vi "CODMn通讯.vi"() -> ()   [LabVIEW 2016, in "斯坦道CODMn.lvlib"]
uses:
  <vilib>/Utility/error.llb/DialogType.ctl
  <vilib>/NI/Modbus Library/API/Wrapper/Create TCP Slave.vi
  <vilib>/NI/Modbus Library/API/slave/Modbus Slave.lvclass
  <vilib>/Plasmionique/MB Master/MB_Master/MB_Master.lvclass
  <vilib>/Plasmionique/MB Master/MB Master.lvlib
  <vilib>/Utility/config.llb/NI_LVConfig.lvlib
  <vilib>/NI/Modbus Library/API/Wrapper/API Main.lvlib
panel:
  out "codm程序更新":bool=TRUE
  in  "读取数据":bool
  in  "释放串口":bool
  in  "打开串口":bool
  out "队列中元素数量":i32
  out "元素":cluster{"命令":string}[](array[cluster])
  out "待处理插入数量":i32
  out "读取公式":u16[](array[numeric])
  out "读取参数":u16[](array[numeric])
  out "数据存储":u16[](array[numeric])
  out "温度":bool[](array[boolean])
  out "M输出点":bool[](array[boolean])
  out "ORP、时间":u16[](array[numeric])
  out "测量状态":u16[](array[numeric])
  out "通讯状态":bool
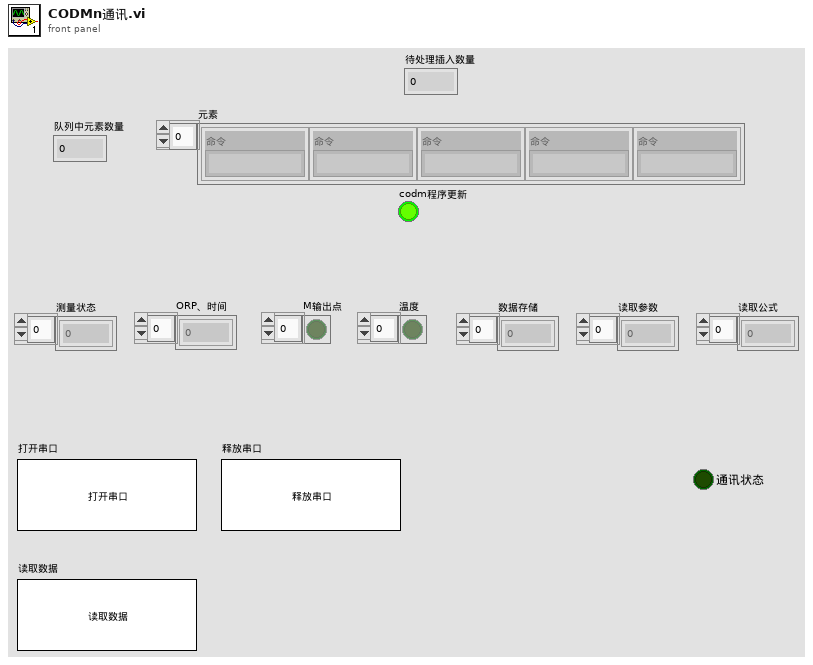
[diagram p1: front panel]
types:
  T1 = typedef "CODMn交互.ctl" = cluster{"COD浓度（mg/L)":dbl, "水样启动时间":timestamp, "加标回收启动时间":timestamp, "CODMn工作状态":enum16{"空闲", "水样测试", "标样核查", "零点核查", "跨度核查", "空白测试", "平行样测试", "加标回收", "空白校准", "标样校准", "初始化（清洗）"}, "多列列表框":i32, "平台试剂余量百分比":sgl, "关键参数":cluster{"测量量程":dbl, "测量精度":dbl, "测量间隔":dbl, "消解温度":dbl, "消解时长":dbl, "空白校准时间":timestamp, "曲线截距":dbl, "曲线斜率":dbl, "测量检出限":dbl, "测量信号值":dbl, "线性相关系数":dbl, "二次多项式系数":dbl, "标样校准时间":timestamp, "稀释倍数":dbl, "三项式系数":dbl, "空白标定系数":dbl, "量程系数":dbl, "F0/ORPA":dbl, "F1/ORPB":dbl, "F2/ORPK":dbl, "F3":dbl, "F4":dbl, "F5":dbl, "F6":dbl, "F7":dbl, "X0/滴定数":dbl, "量程":dbl}, "关键参数改变":bool, "校准信息":cluster{"低标液1浓度":dbl, "低标液1信号值":dbl, "低标液1启用":u16, "低标液2浓度":dbl, "低标液2信号值":dbl, "低标液2启用":u16, "低标液3浓度":dbl, "低标液3信号值":dbl, "低标液3启用":u16, "低标液4浓度":dbl, "低标液4信号值":dbl, "低标液4启用":u16, "低标液5浓度":dbl, "低标液5信号值":dbl, "低标液5启用":u16, "高标液1浓度":dbl, "高标液1信号值":dbl, "高标液1启用":u16, "高标液2浓度":dbl, "高标液2信号值":dbl, "高标液2启用":u16, "高标液3浓度":dbl, "高标液3信号值":dbl, "高标液3启用":u16, "高标液4浓度":dbl, "高标液4信号值":dbl, "高标液4启用":u16, "高标液5浓度":dbl, "高标液5信号值":dbl, "高标液5启用":u16}, "校准信息改变":bool}
  T2 = cluster{"测量模式":enum16{"水样测量", "标样核查", "零点核查", "跨度核查", "空白测试", "加标回收", "平行样", "校零", "校标"}}
  T3 = cluster{"命令":string, "测量模式":enum16{"水样测量", "标样核查", "零点核查", "跨度核查", "空白测试", "加标回收", "平行样", "校零", "校标"}, "CODMn量程切换":enum32{"H", "L", "AUTO"}}
  T4 = typedef "NI_LVConfig.lvlib/Config Data RefNum.ctl" = refnum<k1>
  T5 = enum16{"空闲", "水样测试", "标样核查", "零点核查", "跨度核查", "空白测试", "平行样测试", "质控样", "空白校准", "标样校准", "加标回收"}
  T6 = cluster{"测量量程":dbl, "测量精度":dbl, "测量间隔":dbl, "消解温度":dbl, "消解时长":dbl, "空白校准时间":timestamp, "曲线截距":dbl, "曲线斜率":dbl, "测量检出限":dbl, "测量信号值":dbl, "线性相关系数":dbl, "二次多项式系数":dbl, "标样校准时间":timestamp, "稀释倍数":dbl, "三项式系数":dbl, "空白标定系数":dbl, "量程系数":dbl, "F0/ORPA":dbl, "F1/ORPB":dbl, "F2/ORPK":dbl, "F3":dbl, "F4":dbl, "F5":dbl, "F6":dbl, "F7":dbl, "X0/滴定数":dbl, "量程":dbl}
  T7 = cluster{"低标液1浓度":dbl, "低标液1信号值":dbl, "低标液1启用":u16, "低标液2浓度":dbl, "低标液2信号值":dbl, "低标液2启用":u16, "低标液3浓度":dbl, "低标液3信号值":dbl, "低标液3启用":u16, "低标液4浓度":dbl, "低标液4信号值":dbl, "低标液4启用":u16, "低标液5浓度":dbl, "低标液5信号值":dbl, "低标液5启用":u16, "高标液1浓度":dbl, "高标液1信号值":dbl, "高标液1启用":u16, "高标液2浓度":dbl, "高标液2信号值":dbl, "高标液2启用":u16, "高标液3浓度":dbl, "高标液3信号值":dbl, "高标液3启用":u16, "高标液4浓度":dbl, "高标液4信号值":dbl, "高标液4启用":u16, "高标液5浓度":dbl, "高标液5信号值":dbl, "高标液5启用":u16}
  T8 = typedef "DialogType.ctl" = u16
  T9 = enum16{"水样测量", "标样核查", "零点核查", "跨度核查", "空白测试", "加标回收", "平行样", "校零", "校标"}
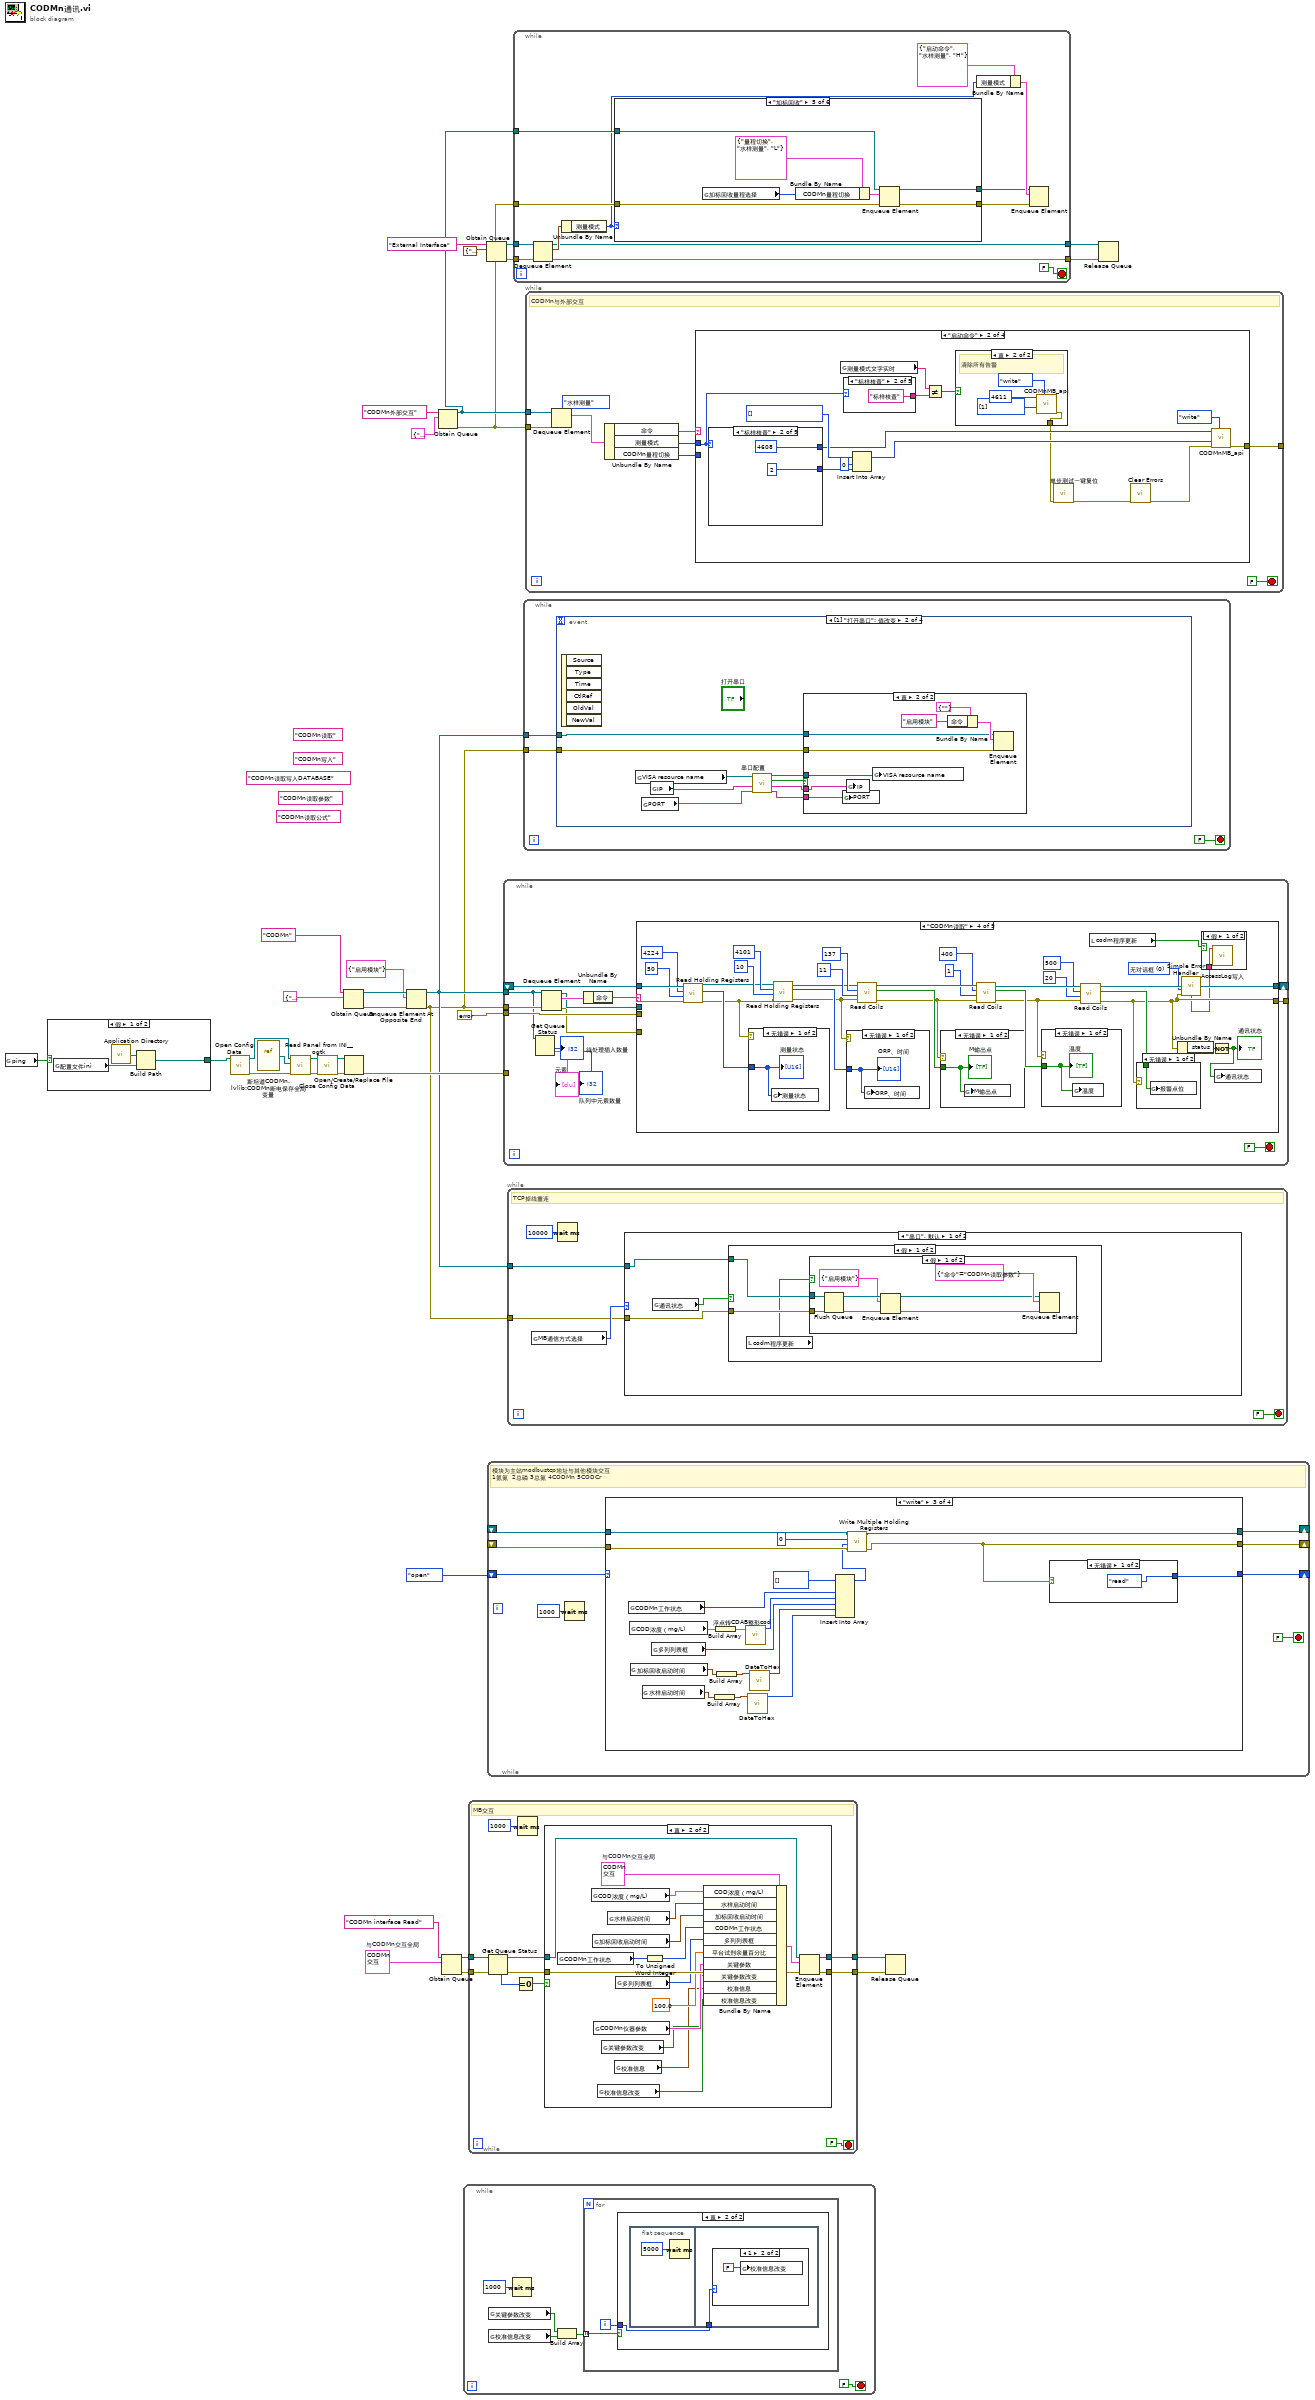
[diagram p0: block diagram]
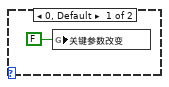
[diagram p3: hidden frame]
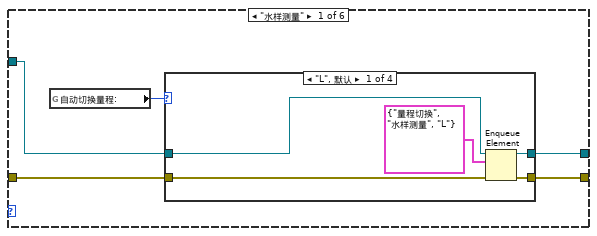
[diagram p5: hidden frame]
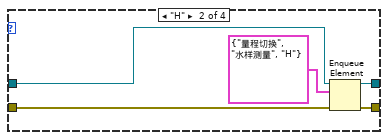
[diagram p6: hidden frame]
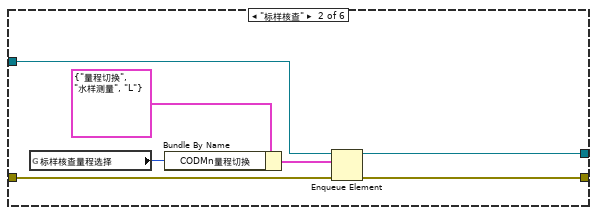
[diagram p9: hidden frame]
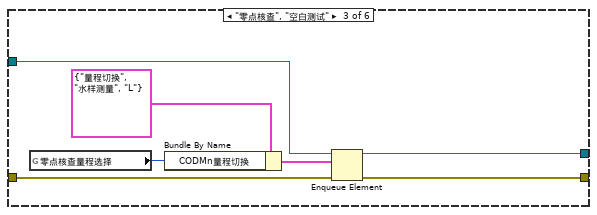
[diagram p10: hidden frame]
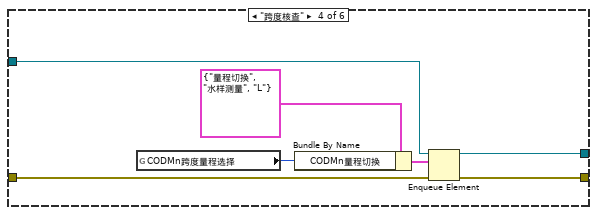
[diagram p11: hidden frame]
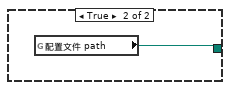
[diagram p13: hidden frame]
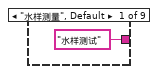
[diagram p16: hidden frame]
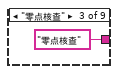
[diagram p17: hidden frame]
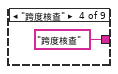
[diagram p18: hidden frame]
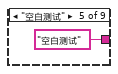
[diagram p19: hidden frame]
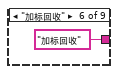
[diagram p20: hidden frame]
diagram:
  w2 = T1 {"COD浓度（mg/L)"=0.0, "水样启动时间"=timestamp(0 s since 1904-01-01), "加标回收启动时间"=timestamp(0 s since 1904-01-01), "CODMn工作状态"=enum."空闲", "多列列表框"=0, "平台试剂余量百分比"=0.0, "关键参数"={"测量量程"=0.0, "测量精度"=0.0, "测量间隔"=0.0, "消解温度"=0.0, "消解时长"=0.0, "空白校准时间"=timestamp(0 s since 1904-01-01), "曲线截距"=0.0, "曲线斜率"=0.0, "测量检出限"=0.0, "测量信号值"=0.0, "线性相关系数"=0.0, "二次多项式系数"=0.0, "标样校准时间"=timestamp(0 s since 1904-01-01), "稀释倍数"=0.0, "三项式系数"=0.0, "空白标定系数"=0.0, "量程系数"=0.0, "F0/ORPA"=0.0, "F1/ORPB"=0.0, "F2/ORPK"=0.0, "F3"=0.0, "F4"=0.0, "F5"=0.0, "F6"=0.0, "F7"=0.0, "X0/滴定数"=0.0, "量程"=0.0}, "关键参数改变"=FALSE, "校准信息"={"低标液1浓度"=0.0, "低标液1信号值"=0.0, "低标液1启用"=0, "低标液2浓度"=0.0, "低标液2信号值"=0.0, "低标液2启用"=0, "低标液3浓度"=0.0, "低标液3信号值"=0.0, "低标液3启用"=0, "低标液4浓度"=0.0, "低标液4信号值"=0.0, "低标液4启用"=0, "低标液5浓度"=0.0, "低标液5信号值"=0.0, "低标液5启用"=0, "高标液1浓度"=0.0, "高标液1信号值"=0.0, "高标液1启用"=0, "高标液2浓度"=0.0, "高标液2信号值"=0.0, "高标液2启用"=0, "高标液3浓度"=0.0, "高标液3信号值"=0.0, "高标液3启用"=0, "高标液4浓度"=0.0, "高标液4信号值"=0.0, "高标液4启用"=0, "高标液5浓度"=0.0, "高标液5信号值"=0.0, "高标液5启用"=0}, "校准信息改变"=FALSE}  # 与CODMn交互全局
  (unwired) "CODMn读取公式" ("名称（未命名）")
  (unwired) "CODMn读取写入DATABASE" ("名称（未命名）")
  (unwired) "CODMn读取参数" ("名称（未命名）")
  (unwired) "CODMn读取" ("名称（未命名）")
  (unwired) "CODMn写入" ("名称（未命名）")
  n1 = global read "CODMN外部API.vi" "ping"() -> (w17:bool)
  n2 = case shown="假" w17 {
    tunnel: [w36 w39] -> w16
    frame False {
      n3 = global read "COD内部交互全局.vi" "配置文件ini"() -> (w38:string)
      n4 = call <vilib>:"Application Directory.vi"() -> ("Application Directory"=w37:path)
      n5 = Build Path(base path=w37, name or relative path=w38) -> (appended path=w36:path)
    }
    frame True {
      n6 = global read "CODMN外部API.vi" "配置文件 path"() -> (w39:path)
    }
  }
  n7 = call <vilib>:"Open Config Data.vi"("configuration file path"=w16) -> ("error out"=w27:errorcluster, "refnum"=w30:T4)  [unwired: 8 in, 1 out]
  n8 = vi-ref "斯坦道CODMn.lvlib:CODMn断电保存全局变量.vi"() -> (w29:refnum<vi>)
  n9 = call <userlib>:"Read Panel from INI__ogtk.vi"("error in (no error)"=w27, "VI ref"=w29, "refnum"=w30) -> ("error out"=w26:errorcluster, "refnum out"=w28:T4)  [unwired: 7 in]
  n10 = call <vilib>:"Close Config Data.vi"("error in (no error)"=w26, "refnum"=w28) -> ("error out"=w25:errorcluster, "file path"=w24:path)  [unwired: 8 in]
  n11 = Obtain Queue(name (unnamed)="CODMn", element data type=cluster{"命令":string} {"命令"="启用模块"} ("元素")) -> (queue out=w33:refnum<queue>, error out=w32:errorcluster)  [unwired: 3 in, 1 out]
  n12 = Open/Create/Replace File(file path (use dialog)=w24, error in=w25) -> (error out=w23:errorcluster)  [unwired: 4 in, 2 out]
  n13 = Enqueue Element At Opposite End(queue=w33, element=cluster{"命令":string} {"命令"="启用模块"} ("元素"), error in (no error)=w32) -> (queue out=w21:refnum<queue>, error out=w20:errorcluster)  [unwired: 1 in, 1 out]
  n14 = Obtain Queue(name (unnamed)="CODMn外部交互" ("名称（未命名）"), element data type=T3 {"命令"="启动命令", "测量模式"=enum."水样测量", "CODMn量程切换"=enum."AUTO"} ("元素")) -> (queue out=w11:refnum<queue>, error out=w10:errorcluster)  [unwired: 3 in, 1 out]
  n15 = Obtain Queue(name (unnamed)="CODMn interface Read" ("写入方名称"), element data type=w2) -> (queue out=w6:refnum<queue>, error out=w5:errorcluster)  [unwired: 3 in, 1 out]
  n16 = while {
    stop <- FALSE stop-if-true
    n17 = global read "CODMn断电保存全局变量.vi" "关键参数改变"() -> (w43:bool)
    n18 = global read "CODMn断电保存全局变量.vi" "校准信息改变"() -> (w42:bool)
    n19 = Wait (ms)(milliseconds to wait=u32 1000 ("等待时间（毫秒）")) -> ()  [unwired: 1 out]
    n20 = Build Array(w43, w42) -> (w41:bool[])
    n21 = for {
      tunnel: w41 -> [w46] mode=indexing
      i -> [w45]
      n22 = case shown="真" w46 {
        tunnel: w45 -> [_ w47]
        frame False {
        }
        frame True {
          n23 = flat-sequence {
            tunnel: w47 -> [w49]
            frame #0 {
              n24 = Wait (ms)(milliseconds to wait=u32 5000 ("等待时间（毫秒）")) -> ()  [unwired: 1 out]
            }
            frame #1 {
              n25 = case shown="1" w49 {
                frame 0, Default {
                  n26 = global write "CODMn断电保存全局变量.vi" "关键参数改变"(FALSE ("关键参数改变")) -> ()
                }
                frame 1 {
                  n27 = global write "CODMn断电保存全局变量.vi" "校准信息改变"(FALSE ("关键参数改变")) -> ()
                }
              }
            }
          }
        }
      }
    }
  }
  n28 = while {
    tunnel: w6 -> [w60]
    tunnel: w5 -> [w53]
    tunnel: [w59] -> w4
    tunnel: [w58] -> w3
    stop <- FALSE stop-if-true
    # "MB交互"
    n29 = Get Queue Status(queue=w60, error in (no error)=w53) -> (queue out=w56:refnum<queue>, error out=w52:errorcluster, # elements in queue=w55:i32)  [unwired: 1 in, 5 out]
    n30 = Equal To 0?(x=w55) -> (x = 0?=w54:bool)
    n31 = Wait (ms)(milliseconds to wait=u32 1000 ("等待时间（毫秒）")) -> ()  [unwired: 1 out]
    n32 = case shown="真" w54 {
      tunnel: w56 -> [w63 w80]
      tunnel: w52 -> [w62 w79]
      tunnel: [w63 w78] -> w59
      tunnel: [w62 w77] -> w58
      frame False {
      }
      frame True {
        w76 = T1 {"COD浓度（mg/L)"=0.0, "水样启动时间"=timestamp(0 s since 1904-01-01), "加标回收启动时间"=timestamp(0 s since 1904-01-01), "CODMn工作状态"=enum."空闲", "多列列表框"=0, "平台试剂余量百分比"=0.0, "关键参数"={"测量量程"=0.0, "测量精度"=0.0, "测量间隔"=0.0, "消解温度"=0.0, "消解时长"=0.0, "空白校准时间"=timestamp(0 s since 1904-01-01), "曲线截距"=0.0, "曲线斜率"=0.0, "测量检出限"=0.0, "测量信号值"=0.0, "线性相关系数"=0.0, "二次多项式系数"=0.0, "标样校准时间"=timestamp(0 s since 1904-01-01), "稀释倍数"=0.0, "三项式系数"=0.0, "空白标定系数"=0.0, "量程系数"=0.0, "F0/ORPA"=0.0, "F1/ORPB"=0.0, "F2/ORPK"=0.0, "F3"=0.0, "F4"=0.0, "F5"=0.0, "F6"=0.0, "F7"=0.0, "X0/滴定数"=0.0, "量程"=0.0}, "关键参数改变"=FALSE, "校准信息"={"低标液1浓度"=0.0, "低标液1信号值"=0.0, "低标液1启用"=0, "低标液2浓度"=0.0, "低标液2信号值"=0.0, "低标液2启用"=0, "低标液3浓度"=0.0, "低标液3信号值"=0.0, "低标液3启用"=0, "低标液4浓度"=0.0, "低标液4信号值"=0.0, "低标液4启用"=0, "低标液5浓度"=0.0, "低标液5信号值"=0.0, "低标液5启用"=0, "高标液1浓度"=0.0, "高标液1信号值"=0.0, "高标液1启用"=0, "高标液2浓度"=0.0, "高标液2信号值"=0.0, "高标液2启用"=0, "高标液3浓度"=0.0, "高标液3信号值"=0.0, "高标液3启用"=0, "高标液4浓度"=0.0, "高标液4信号值"=0.0, "高标液4启用"=0, "高标液5浓度"=0.0, "高标液5信号值"=0.0, "高标液5启用"=0}, "校准信息改变"=FALSE}  # 与CODMn交互全局
        n33 = global read "COD测量模式全局.vi" "CODMn工作状态"() -> (w73:T5)
        n34 = global read "COD浓度全局变量.vi" "COD浓度（mg/L)"() -> (w68:dbl)
        n35 = global read "COD测量模式全局.vi" "加标回收启动时间"() -> (w72:timestamp)
        n36 = global read "CODMn断电保存全局变量.vi" "CODMn仪器参数"() -> (w75:T6)
        n37 = global read "CODMn断电保存全局变量.vi" "校准信息改变"() -> (w65:bool)
        n38 = global read "CODMn断电保存全局变量.vi" "关键参数改变"() -> (w66:bool)
        n39 = global read "COD测量模式全局.vi" "水样启动时间"() -> (w71:timestamp)
        n40 = global read "CODMn断电保存全局变量.vi" "校准信息"() -> (w64:T7)
        n41 = global read "运行时序全局变量.vi" "多列列表框"() -> (w69:i32)
        n42 = To Unsigned Word Integer(number=w73) -> (unsigned 16bit integer=w74:u16)
        n43 = Bundle By Name(cluster=w76, "COD浓度（mg/L)"=w68, "水样启动时间"=w71, "加标回收启动时间"=w72, "CODMn工作状态"=w74, "多列列表框"=w69, "平台试剂余量百分比"=sgl 100.0, "关键参数"=w75, "关键参数改变"=w66, "校准信息"=w64, "校准信息改变"=w65) -> (w67:T1)
        n44 = Enqueue Element(queue=w80, element=w67, error in (no error)=w79) -> (queue out=w78:refnum<queue>, error out=w77:errorcluster)  [unwired: 1 in, 1 out]
      }
    }
  }
  n45 = Obtain Queue(name (unnamed)="External Interface" ("名称（未命名）"), element data type=T2 {"测量模式"=enum."水样测量"} ("启动测量模式")) -> (queue out=w13:refnum<queue>, error out=w12:errorcluster)  [unwired: 3 in, 1 out]
  n46 = while {
    shift-right: [w86] -> _
    shift-left: _ -> [w88]
    shift-right: [w85] -> _
    shift-left: _ -> [w87]
    shift-right: [w82] -> _
    shift-left: enum16{"open", "read", "write", "close"}."open" -> [w83]
    stop <- FALSE stop-if-true
    # "模块为主站modbustcp地址与其他模块交互\n1氨氮  2总磷 3总氮 4CODMn 5CODCr"
    n47 = Wait (ms)(milliseconds to wait=u32 1000 ("等待时间（毫秒）")) -> ()  [unwired: 1 out]
    n48 = case shown="\"write\"" w83 {
      selector: w83 -> [w97 _ _ _]
      tunnel: w88 -> [w91 w105 w128 w134]
      tunnel: w87 -> [w90 w104 w125 w133]
      tunnel: [w94 w101 w127 w134] -> w86
      tunnel: [w93 w100 w126 w136] -> w85
      tunnel: [w96 w108 w129 enum16{"open", "read", "write", "close"}."open"] -> w82
      frame "open", Default {
        n49 = call-dynamic "Shutdown.vi"("error in"=w90, "Modbus slave in"=w91) -> ("error out"=w89:errorcluster)  [unwired: 9 in]
        n50 = call <vilib>:"Clear Errors.vi"("error in (no error)"=w89) -> ("error out"=w92:errorcluster)  [unwired: 5 in, 1 out]
        n51 = call-poly <vilib>:"Create Modbus Instance.vi"("error in"=w92, "port (502)"=u16 4) -> ("error out"=w93:errorcluster, "TCP slave instance"=w94:refnum<class "Modbus Slave.lvclass">)  [unwired: 8 in]
        n52 = case shown="错误" w93 {
          tunnel: w97 -> [_ w99]
          tunnel: [enum16{"open", "read", "write", "close"}."write" w99] -> w96
          frame No Error {
          }
          frame Error {
          }
        }
      }
      frame "read" {
        n53 = call-dynamic <vilib>:"Read Holding Registers.vi"("error in"=w104, "number of inputs"=u16 1, "starting address"=u16 257, "Modbus slave in"=w105) -> ("error out"=w100:errorcluster, "register values"=w103:u16[], "Modbus slave out"=w101:refnum<class "Modbus Slave.lvclass">)  [unwired: 5 in]
        n54 = Index Array(array=w103) -> (element=w102:u16)  [unwired: 1 in]
        n55 = global write "CODMN外部API.vi" "CODMn状态"(w102) -> ()
        n56 = case shown="无错误" w100 {
          tunnel: [enum16{"open", "read", "write", "close"}."write" enum16{"open", "read", "write", "close"}."close"] -> w108
          frame No Error {
          }
          frame Error {
          }
        }
      }
      frame "write" {
        n57 = global read "COD测量模式全局.vi" "CODMn工作状态"() -> (w115:T5)
        n58 = global read "COD浓度全局变量.vi" "COD浓度（mg/L)"() -> (w117:dbl)
        n59 = global read "COD测量模式全局.vi" "加标回收启动时间"() -> (w120:timestamp)
        n60 = global read "COD测量模式全局.vi" "水样启动时间"() -> (w122:timestamp)
        n61 = global read "运行时序全局变量.vi" "多列列表框"() -> (w119:i32)
        n62 = Build Array(w122) -> (w121:timestamp[])
        n63 = Build Array(w117) -> (w116:dbl[])
        n64 = Build Array(w120) -> (w113:timestamp[])
        n65 = call "浮点转CDAB整形cod.vi"("浮点数"=w116) -> ("CDAB整形输出"=w118:u16[])  [unwired: 10 in]
        n66 = call "DateToHex.vi"("DATE"=w121) -> ("数组"=w124:u16[])  [unwired: 10 in]
        n67 = call "DateToHex.vi"("DATE"=w113) -> ("数组"=w123:u16[])  [unwired: 10 in]
        n68 = Insert Into Array(array=u16[] [] ("values"), new element #1=w115, new element #2=w118, new element #3=w119, new element #4=w123, new element #5=w124) -> (w112:u16[])  [unwired: 1 in]
        n69 = call-dynamic "Write Multiple Holding Registers.vi"("error in"=w125, "registers to write"=w112, "starting address"=u16 0, "Modbus slave in"=w128) -> ("error out"=w126:errorcluster, "Modbus slave out"=w127:refnum<class "Modbus Slave.lvclass">)  [unwired: 6 in]
        n70 = case shown="无错误" w126 {
          tunnel: [enum16{"open", "read", "write", "close"}."read" enum16{"open", "read", "write", "close"}."close"] -> w129
          frame No Error {
          }
          frame Error {
          }
        }
      }
      frame "close" {
        n71 = call-dynamic "Shutdown.vi"("error in"=w133, "Modbus slave in"=w134) -> ("error out"=w132:errorcluster)  [unwired: 9 in]
        n72 = call <vilib>:"Clear Errors.vi"("error in (no error)"=w132) -> ("error out"=w136:errorcluster)  [unwired: 5 in, 1 out]
      }
    }
  }
  n73 = while {
    tunnel: w21 -> [w142]
    tunnel: w20 -> [w149]
    tunnel: [w143] -> _
    shift-right: [w146] -> _
    shift-left: _ -> [w145]
    tunnel: errorcluster {"status"=FALSE, "code"=0, "source"=""} ("error out") -> [w144]
    tunnel: w23 -> [_]
    stop <- FALSE stop-if-true
    n74 = Get Queue Status(queue=w142) -> (# pending insert=→"待处理插入数量":i32, # elements in queue=→"队列中元素数量":i32, elements=→"元素":cluster{"命令":string}[])  [unwired: 2 in, 5 out]
    n75 = Dequeue Element(queue=w142, error in (no error)=w149) -> (queue out=w138:refnum<queue>, element=w148:cluster{"命令":string}, error out=w137:errorcluster)  [unwired: 1 in, 1 out]
    n76 = Unbundle By Name(w148) -> ("命令"=w147:string)
    n77 = case shown="\"CODMn读取\"" w147 {
      tunnel: [w152 w157 w169 w180 w213 w222 w239 w246 w253] -> w146
      tunnel: [w151 w154 w170 w175 w211 w221 w238 w245 w252] -> w143
      tunnel: w145 -> [w152 _ _ w204 w217 w231 w242 w250 w256]
      tunnel: w144 -> [w151 w158 w171 w203 w214 w230 w241 w249 w254]
      tunnel: w138 -> [_ w156 _ _ _ _ _ _ _]
      tunnel: w137 -> [_ w155 _ _ _ _ _ _ _]
      frame Default {
      }
      frame "启用模块" {
        n78 = call "CODMnMB_api.vi"("STEP"=enum16{"open", "read", "write", "close"}."open", "Error in"=w158) -> ("error out"=w154:errorcluster, "MB session out"=w157:refnum<class "MB_Master.lvclass">)  [unwired: 7 in, 1 out]
        n79 = case shown="无错误" w154 {
          tunnel: w156 -> [w164 _]
          tunnel: w155 -> [w163 _]
          frame No Error {
            n80 = global read "COD内部交互全局.vi" "序列号:"() -> (w162:string)
            n81 = Empty String/Path?(string/path=w162) -> (empty?=w161:bool)
            n82 = Not(x=w161) -> (.not. x?=w160:bool)
            n83 = case shown="真" w160 {
              tunnel: w164 -> [_ w167]
              tunnel: w163 -> [_ w166]
              frame False {
              }
              frame True {
                # "发货调试版用"
                n84 = Enqueue Element(queue=w167, element=cluster{"命令":string} {"命令"="CODMn序列号写入"} ("元素"), error in (no error)=w166) -> ()  [unwired: 1 in, 3 out]
              }
            }
          }
          frame Error {
          }
        }
        n85 = global write "COD浓度全局变量.vi" "MB session in"(w157) -> ()
        n86 = local write "codm程序更新"(FALSE ("codm程序更新")) -> ()
      }
      frame "停用模块" {
        n87 = call "CODMnMB_api.vi"("STEP"=enum16{"open", "read", "write", "close"}."close", "Error in"=w171) -> ("error out"=w170:errorcluster, "MB session out"=w169:refnum<class "MB_Master.lvclass">)  [unwired: 7 in, 1 out]
        "codm程序更新" <- TRUE
      }
      frame "CODMn读取" {
        w176 = T8 0 items=["无对话框", "确定信息", "继续或停止信息", "确定信息＋警告", "继续/停止+警告"] ("type of dialog (OK msg:1)")
        n88 = call <vilib>:"Read Holding Registers.vi"("error in (no error)"=w203, "quantity"=u16 50 ("number of holding registers"), "starting address"=u16 4224, "MB session in"=w204) -> ("error out"=w194:errorcluster, "Registers"=w200:u16[], "MB session out"=w195:refnum<class "MB_Master.lvclass">)  [unwired: 5 in]
        n89 = case shown="无错误" w194 {
          tunnel: w200 -> [w210 _]
          frame No Error {
            n90 = global write "COD内部交互全局.vi" "测量状态"(w210) -> ()
            "测量状态" <- w210
          }
          frame Error {
          }
        }
        n91 = call <vilib>:"Read Holding Registers.vi"("error in (no error)"=w194, "quantity"=u16 10, "starting address"=u16 4101, "MB session in"=w195) -> ("error out"=w190:errorcluster, "Registers"=w193:u16[], "MB session out"=w192:refnum<class "MB_Master.lvclass">)  [unwired: 5 in]
        n92 = case shown="无错误" w190 {
          tunnel: w193 -> [w209 _]
          frame No Error {
            n93 = global write "COD内部交互全局.vi" "ORP、时间"(w209) -> ()
            "ORP、时间" <- w209
          }
          frame Error {
          }
        }
        n94 = call <vilib>:"Read Coils.vi"("error in (no error)"=w190, "quantity"=u16 11, "starting address"=u16 137, "MB session in"=w192) -> ("error out"=w188:errorcluster, "Coils"=w189:bool[], "MB session out"=w191:refnum<class "MB_Master.lvclass">)  [unwired: 5 in]
        n95 = case shown="无错误" w188 {
          tunnel: w189 -> [w208 _]
          frame No Error {
            n96 = global write "COD内部交互全局.vi" "M输出点"(w208) -> ()
            "M输出点" <- w208
          }
          frame Error {
          }
        }
        n97 = call <vilib>:"Read Coils.vi"("error in (no error)"=w188, "quantity"=u16 1, "starting address"=u16 400, "MB session in"=w191) -> ("error out"=w181:errorcluster, "Coils"=w185:bool[], "MB session out"=w182:refnum<class "MB_Master.lvclass">)  [unwired: 5 in]
        n98 = case shown="无错误" w181 {
          tunnel: w185 -> [w207 _]
          frame No Error {
            n99 = global write "COD内部交互全局.vi" "温度"(w207) -> ()
            "温度" <- w207
          }
          frame Error {
          }
        }
        n100 = call <vilib>:"Read Coils.vi"("error in (no error)"=w181, "quantity"=u16 20, "starting address"=u16 500, "MB session in"=w182) -> ("error out"=w175:errorcluster, "Coils"=w177:bool[], "MB session out"=w180:refnum<class "MB_Master.lvclass">)  [unwired: 5 in]
        n101 = local read "codm程序更新"() -> (w173:bool)
        n102 = case shown="无错误" w175 {
          tunnel: w177 -> [w206 _]
          frame No Error {
            n103 = global write "COD内部交互全局.vi" "报警点位"(w206) -> ()
          }
          frame Error {
          }
        }
        n104 = Unbundle By Name(w175) -> ("status"=w184:bool)
        n105 = call <vilib>:"Simple Error Handler.vi"("type of dialog (OK msg:1)"=w176, "error in (no error)"=w175) -> ("message"=w174:string)  [unwired: 3 in, 4 out]
        n106 = case shown="假" w173 {
          tunnel: w174 -> [w205 _]
          frame False {
            n107 = call "AccessLog写入.vi"("Log"=w205) -> ()  [unwired: 11 in]
          }
          frame True {
          }
        }
        n108 = Not(x=w184) -> (.not. x?=w183:bool)
        "通讯状态" <- w183
        n109 = global write "COD内部交互全局.vi" "通讯状态"(w183) -> ()
      }
      frame "CODMn读取写入DATABASE" {
        n110 = call <vilib>:"Read Holding Registers.vi"("error in (no error)"=w214, "quantity"=u16 10 ("number of holding registers"), "starting address"=u16 4101, "MB session in"=w217) -> ("error out"=w211:errorcluster, "Registers"=w212:u16[], "MB session out"=w213:refnum<class "MB_Master.lvclass">)  [unwired: 5 in]
        n111 = case shown="无错误" w211 {
          tunnel: w212 -> [w219 _]
          frame No Error {
            n112 = global write "COD内部交互全局.vi" "数据存储"(w219) -> ()
            n113 = global write "COD内部交互全局.vi" "读取写入data"(TRUE ("读取参数显示")) -> ()
            "数据存储" <- w219
          }
          frame Error {
          }
        }
      }
      frame "CODMn读取参数" {
        n114 = call <vilib>:"Read Holding Registers.vi"("error in (no error)"=w230, "quantity"=u16 35 ("number of holding registers"), "starting address"=u16 4272, "MB session in"=w231) -> ("error out"=w225:errorcluster, "Registers"=w227:u16[], "MB session out"=w226:refnum<class "MB_Master.lvclass">)  [unwired: 5 in]
        n115 = case shown="无错误" w225 {
          tunnel: w227 -> [w235 _]
          frame No Error {
            n116 = global write "COD内部交互全局.vi" "读取参数"(w235) -> ()
            n117 = global write "COD内部交互全局.vi" "读取参数显示"(TRUE ("读取参数显示")) -> ()
            "读取参数" <- w235
          }
          frame Error {
          }
        }
        n118 = call <vilib>:"Read Holding Registers.vi"("error in (no error)"=w225, "quantity"=u16 4, "starting address"=u16 5596, "MB session in"=w226) -> ("error out"=w221:errorcluster, "Registers"=w220:u16[], "MB session out"=w222:refnum<class "MB_Master.lvclass">)  [unwired: 5 in]
        n119 = case shown="无错误" w221 {
          tunnel: w220 -> [w233 _]
          frame No Error {
            n120 = global write "COD内部交互全局.vi" "读取浮台参数"(w233) -> ()
            n121 = global write "COD内部交互全局.vi" "读取浮台参数显示"(TRUE ("读取参数显示")) -> ()
          }
          frame Error {
          }
        }
      }
      frame "CODMn读取公式" {
        n122 = call <vilib>:"Read Holding Registers.vi"("error in (no error)"=w241, "quantity"=u16 94 ("number of holding registers"), "starting address"=u16 4616, "MB session in"=w242) -> ("error out"=w238:errorcluster, "Registers"=w240:u16[], "MB session out"=w239:refnum<class "MB_Master.lvclass">)  [unwired: 5 in]
        n123 = case shown="无错误" w238 {
          tunnel: w240 -> [w244 _]
          frame No Error {
            n124 = global write "COD内部交互全局.vi" "读取公式"(w244) -> ()
            n125 = global write "COD内部交互全局.vi" "读取公式显示"(TRUE ("读取参数显示")) -> ()
            "读取公式" <- w244
          }
          frame Error {
          }
        }
      }
      frame "CODMn序列号写入" {
        n126 = global read "COD内部交互全局.vi" "序列号:"() -> (w248:string)
        n127 = call "StringToHex.vi"("STRING"=w248) -> ("数组"=w247:u16[])  [unwired: 10 in]
        n128 = call <vilib>:"Write Multiple Registers.vi"("error in (no error)"=w249, "values"=w247, "starting address"=u16 4298, "MB session in"=w250) -> ("error out"=w245:errorcluster, "MB session out"=w246:refnum<class "MB_Master.lvclass">)  [unwired: 6 in]
      }
      frame "CODMn程序更新" {
        n129 = call <vilib>:"Write Multiple Registers.vi"("error in (no error)"=w254, "values"=u16[] [0], "starting address"=u16 4296, "MB session in"=w256) -> ("error out"=w252:errorcluster, "MB session out"=w253:refnum<class "MB_Master.lvclass">)  [unwired: 6 in]
      }
    }
  }
  n130 = while "While循环" {
    tunnel: w21 -> [w259]
    tunnel: w20 -> [w258]
    stop <- FALSE stop-if-true
    # "TCP掉线重连"
    n131 = global read "CODMn断电保存全局变量.vi" "MB通信方式选择"() -> (w260:enum16{"串口", "TCP"})
    n132 = Wait (ms)(milliseconds to wait=u32 10000 ("等待时间（毫秒）")) -> ()  [unwired: 1 out]
    n133 = case shown="\"串口\", 默认" w260 {
      tunnel: w259 -> [w264 w278]
      tunnel: w258 -> [w263 w277]
      frame "串口", Default {
        n134 = global read "COD内部交互全局.vi" "通讯状态"() -> (w265:bool)
        n135 = case shown="假" w265 {
          tunnel: w264 -> [w268 _]
          tunnel: w263 -> [w267 _]
          frame False {
            n136 = local read "codm程序更新"() -> (w266:bool)
            n137 = case shown="假" w266 {
              tunnel: w268 -> [w273 _]
              tunnel: w267 -> [w272 _]
              frame False {
                n138 = Flush Queue(queue=w273, error in (no error)=w272) -> (queue out=w276:refnum<queue>, error out=w275:errorcluster)  [unwired: 1 out]
                n139 = Enqueue Element(queue=w276, element=cluster{"命令":string} {"命令"="启用模块"} ("元素"), error in (no error)=w275) -> (queue out=w270:refnum<queue>, error out=w269:errorcluster)  [unwired: 1 in, 1 out]
                n140 = Enqueue Element(queue=w270, element=cluster{"命令":string} {"命令"="CODMn读取参数"} ("元素"), error in (no error)=w269) -> ()  [unwired: 1 in, 3 out]
              }
              frame True {
              }
            }
          }
          frame True {
          }
        }
      }
      frame "TCP" {
        n141 = global read "COD浓度全局变量.vi" "MB session in"() -> (w280:refnum<class "MB_Master.lvclass">)
        n142 = property class="MB_Master"(reference=w280) -> ("Properties:Session Valid"=w279:bool)  [unwired: 1 in, 2 out]
        n143 = case shown="假" w279 {
          tunnel: w278 -> [w285 _]
          tunnel: w277 -> [w284 _]
          frame False {
            n144 = Flush Queue(queue=w285, error in (no error)=w284) -> (queue out=w288:refnum<queue>, error out=w287:errorcluster)  [unwired: 1 out]
            n145 = Enqueue Element(queue=w288, element=cluster{"命令":string} {"命令"="启用模块"} ("元素"), error in (no error)=w287) -> (queue out=w282:refnum<queue>, error out=w281:errorcluster)  [unwired: 1 in, 1 out]
            n146 = Enqueue Element(queue=w282, element=cluster{"命令":string} {"命令"="CODMn读取参数"} ("元素"), error in (no error)=w281) -> ()  [unwired: 1 in, 3 out]
          }
          frame True {
          }
        }
      }
    }
  }
  n147 = while {
    tunnel: w13 -> [w301]
    tunnel: w12 -> [w300]
    tunnel: w11 -> [w297]
    tunnel: w10 -> [w296]
    tunnel: [w290] -> w9
    tunnel: [w289] -> w8
    stop <- FALSE stop-if-true
    n148 = Dequeue Element(queue=w301, error in (no error)=w300) -> (queue out=w290:refnum<queue>, element=w298:T2, error out=w289:errorcluster)  [unwired: 1 in, 1 out]
    n149 = Unbundle By Name(w298) -> ("测量模式"=w293:T9)
    n150 = case "条件结构" shown="\"加标回收\"" w293 {
      tunnel: w297 -> [w305 w324 w331 w338 w345 w350]
      tunnel: w296 -> [w303 w323 w330 w337 w344 w349]
      tunnel: [w304 w322 w329 w336 w343 w350] -> w292
      tunnel: [w302 w321 w328 w335 w342 w349] -> w291
      frame "水样测量" {
        n151 = global read "CODMn断电保存全局变量.vi" "自动切换量程:"() -> (w306:enum16{"L", "H", "自动切换测一次", "自动切换测两次"})
        n152 = case shown="\"L\", 默认" w306 {
          tunnel: w305 -> [w310 w316 w317 w320]
          tunnel: [w308 w315 w317 w320] -> w304
          tunnel: w303 -> [w309 w314 w318 w319]
          tunnel: [w307 w313 w318 w319] -> w302
          frame "L", Default {
            n153 = Enqueue Element(queue=w310, element=T3 {"命令"="量程切换", "测量模式"=enum."水样测量", "CODMn量程切换"=enum."L"} ("元素"), error in (no error)=w309) -> (queue out=w308:refnum<queue>, error out=w307:errorcluster)  [unwired: 1 in, 1 out]
          }
          frame "H" {
            n154 = Enqueue Element(queue=w316, element=T3 {"命令"="量程切换", "测量模式"=enum."水样测量", "CODMn量程切换"=enum."H"} ("元素"), error in (no error)=w314) -> (queue out=w315:refnum<queue>, error out=w313:errorcluster)  [unwired: 1 in, 1 out]
          }
          frame "自动切换测一次" {
          }
          frame "自动切换测两次" {
          }
        }
      }
      frame "标样核查" {
        n155 = global read "CODMn断电保存全局变量.vi" "标样核查量程选择"() -> (w326:enum32{"H", "L", "AUTO"})
        n156 = Bundle By Name(cluster=T3 {"命令"="量程切换", "测量模式"=enum."水样测量", "CODMn量程切换"=enum."L"} ("元素"), "CODMn量程切换"=w326) -> (w327:T3)
        n157 = Enqueue Element(queue=w324, element=w327, error in (no error)=w323) -> (queue out=w322:refnum<queue>, error out=w321:errorcluster)  [unwired: 1 in, 1 out]
      }
      frame "零点核查", "空白测试" {
        n158 = global read "CODMn断电保存全局变量.vi" "零点核查量程选择"() -> (w333:enum32{"H", "L", "AUTO"})
        n159 = Bundle By Name(cluster=T3 {"命令"="量程切换", "测量模式"=enum."水样测量", "CODMn量程切换"=enum."L"} ("元素"), "CODMn量程切换"=w333) -> (w332:T3)
        n160 = Enqueue Element(queue=w331, element=w332, error in (no error)=w330) -> (queue out=w329:refnum<queue>, error out=w328:errorcluster)  [unwired: 1 in, 1 out]
      }
      frame "跨度核查" {
        n161 = global read "CODMn断电保存全局变量.vi" "CODMn跨度量程选择"() -> (w340:enum32{"H", "L", "AUTO"})
        n162 = Bundle By Name(cluster=T3 {"命令"="量程切换", "测量模式"=enum."水样测量", "CODMn量程切换"=enum."L"} ("元素"), "CODMn量程切换"=w340) -> (w339:T3)
        n163 = Enqueue Element(queue=w338, element=w339, error in (no error)=w337) -> (queue out=w336:refnum<queue>, error out=w335:errorcluster)  [unwired: 1 in, 1 out]
      }
      frame "加标回收" {
        n164 = global read "CODMn断电保存全局变量.vi" "加标回收量程选择"() -> (w347:enum32{"H", "L", "AUTO"})
        n165 = Bundle By Name(cluster=T3 {"命令"="量程切换", "测量模式"=enum."水样测量", "CODMn量程切换"=enum."L"} ("元素"), "CODMn量程切换"=w347) -> (w346:T3)
        n166 = Enqueue Element(queue=w345, element=w346, error in (no error)=w344) -> (queue out=w343:refnum<queue>, error out=w342:errorcluster)  [unwired: 1 in, 1 out]
      }
      frame Default {
        # "不切换量程"
      }
    }
    n167 = Bundle By Name(cluster=T3 {"命令"="启动命令", "测量模式"=enum."水样测量", "CODMn量程切换"=enum."H"} ("元素"), "测量模式"=w293) -> (w294:T3)
    n168 = Enqueue Element(queue=w292, element=w294, error in (no error)=w291) -> ()  [unwired: 1 in, 3 out]
  }
  n169 = while {
    tunnel: w21 -> [w352]
    tunnel: w20 -> [w351]
    stop <- FALSE stop-if-true
    n170 = event shown="[1] \"打开串口\": 值改变" {
      selector: _ -> [_ _ _ _]
      dyn-events: _ -> [_ _ _ _]
      timeout: _ -> [_ _ _ _]
      tunnel: w352 -> [_ w359 w373 w375]
      tunnel: w351 -> [_ w358 w372 w374]
      event Timeout {
        n171 = event-data() -> ()  [unwired: 1 in, 3 out]
      }
      event "打开串口": Value Change {
        n172 = event-data() -> ()  [unwired: 1 in, 6 out]
        n173 = global read "CODMn断电保存全局变量.vi" "VISA resource name"() -> (w362:refnum<visa-resource-name>)
        n174 = global read "CODMn断电保存全局变量.vi" "PORT"() -> (w354:string)
        n175 = global read "CODMn断电保存全局变量.vi" "IP"() -> (w355:string)
        n176 = call "串口配置.vi"("PORT"=w354, "IP"=w355, "请选择串口:"=w362) -> ("PORT 2"=w356:string, "IP 2"=w357:string, "确认 2"=w360:bool, "VISA资源名称 2"=w361:refnum<visa-resource-name>)  [unwired: 4 in, 1 out]
        n177 = case shown="真" w360 {
          tunnel: w361 -> [_ w370]
          tunnel: w359 -> [_ w366]
          tunnel: w358 -> [_ w365]
          tunnel: w357 -> [_ w364]
          tunnel: w356 -> [_ w363]
          frame False {
          }
          frame True {
            n178 = global write "CODMn断电保存全局变量.vi" "PORT"(w363) -> ()
            n179 = global write "CODMn断电保存全局变量.vi" "IP"(w364) -> ()
            n180 = global write "CODMn断电保存全局变量.vi" "VISA resource name"(w370) -> ()
            n181 = Bundle By Name(cluster=cluster{"命令":string} {"命令"=""} ("元素"), "命令"="启用模块" ("名称（未命名）")) -> (w367:cluster{"命令":string})
            n182 = Enqueue Element(queue=w366, element=w367, error in (no error)=w365) -> ()  [unwired: 1 in, 3 out]
          }
        }
      }
      event "释放串口": Value Change {
        n183 = event-data() -> ()  [unwired: 1 in, 6 out]
        n184 = Enqueue Element(queue=w373, element=cluster{"命令":string} {"命令"="停用模块"} ("元素"), error in (no error)=w372) -> ()  [unwired: 1 in, 3 out]
      }
      event "读取数据": Value Change {
        n185 = event-data() -> ()  [unwired: 1 in, 6 out]
        n186 = Enqueue Element(queue=w375, element=cluster{"命令":string} {"命令"="CODMn读取"} ("元素"), error in (no error)=w374) -> ()  [unwired: 1 in, 3 out]
      }
    }
  }
  n187 = while {
    tunnel: w11 -> [w382]
    tunnel: w10 -> [w381]
    tunnel: [w377] -> _
    stop <- FALSE stop-if-true
    (unwired) T9."水样测量" ("测量模式")
    # "CODMn与外部交互"
    n188 = Dequeue Element(queue=w382, error in (no error)=w381) -> (element=w383:T3)  [unwired: 1 in, 3 out]
    n189 = Unbundle By Name(w383) -> ("命令"=w380:string, "测量模式"=w379:T9, "CODMn量程切换"=w378:enum32{"H", "L", "AUTO"})
    n190 = case shown="\"启动命令\"" w380 {
      tunnel: w379 -> [_ w387 _ _]
      tunnel: w378 -> [_ _ _ w437]
      tunnel: [_ w392 w432 w436] -> w377
      frame "假", Default {
      }
      frame "启动命令" {
        n191 = case shown="\"标样核查\"" w387 {
          tunnel: [u16 4608 ("address") u16 4608 ("address") u16 4608 ("address") u16 4608 ("address") u16 4608 ("address") u16 4608 ("address") u16 4608 ("address") u16 4608 ("address") u16 4608 ("address")] -> w394
          tunnel: [u16 1 ("address") u16 2 ("address") u16 3 ("address") u16 4 ("address") u16 5 ("address") u16 7 ("address") u16 6 ("address") u16 8 ("address") u16 9 ("address")] -> w398
          frame "水样测量" {
          }
          frame "标样核查" {
          }
          frame "零点核查" {
          }
          frame "跨度核查" {
          }
          frame "空白测试" {
          }
          frame "加标回收" {
          }
          frame "平行样" {
          }
          frame "校零" {
            n192 = global write "CODMN外部API.vi" "远程反控校零CODMn"(TRUE ("远程反控校准CODMn")) -> ()
          }
          frame "校标" {
            n193 = global write "CODMN外部API.vi" "远程反控校准CODMn"(TRUE ("远程反控校准CODMn")) -> ()
          }
        }
        n194 = global read "COD测量模式全局.vi" "测量模式文字实时"() -> (w388:string)
        n195 = case shown="\"标样核查\"" w387 {
          tunnel: ["水样测试" ("测量模式") "标样核查" ("测量模式") "零点核查" ("测量模式") "跨度核查" ("测量模式") "空白测试" ("测量模式") "加标回收" ("测量模式") "平行样" ("测量模式") "校零" ("测量模式") "校标" ("测量模式")] -> w389
          frame "水样测量", Default {
          }
          frame "标样核查" {
          }
          frame "零点核查" {
          }
          frame "跨度核查" {
          }
          frame "空白测试" {
          }
          frame "加标回收" {
          }
          frame "平行样" {
          }
          frame "校零" {
          }
          frame "校标" {
          }
        }
        n196 = Insert Into Array(array=u16[] [] ("values"), index=0 ("索引"), new element=w398) -> (w393:u16[])
        n197 = Not Equal?(x=w388, y=w389) -> (x != y?=w386:bool)
        n198 = case shown="真" w386 {
          tunnel: [_ w399] -> w385
          frame False {
          }
          frame True {
            # "清除所有告警"
            n199 = call "CODMnMB_api.vi"("STEP"=enum16{"open", "read", "write", "close"}."write", "values"=u16[] [1], "starting address"=u16 4611) -> ("error out"=w399:errorcluster)  [unwired: 6 in, 2 out]
          }
        }
        n200 = call "单步测试一键复位.vi"("Error in"=w385) -> ("error out"=w391:errorcluster)  [unwired: 10 in]
        n201 = call <vilib>:"Clear Errors.vi"("error in (no error)"=w391) -> ("error out"=w390:errorcluster)  [unwired: 5 in, 1 out]
        n202 = call "CODMnMB_api.vi"("STEP"=enum16{"open", "read", "write", "close"}."write", "Error in"=w390, "values"=w393, "starting address"=w394) -> ("error out"=w392:errorcluster)  [unwired: 5 in, 2 out]
      }
      frame "停止命令" {
        n203 = call "CODMnMB_api.vi"("STEP"=enum16{"open", "read", "write", "close"}."write", "values"=u16[] [11], "starting address"=u16 4608) -> ("error out"=w432:errorcluster)  [unwired: 6 in, 2 out]
      }
      frame "量程切换" {
        n204 = case shown="\"H\"" w437 {
          tunnel: [u16[] [1] ("values") u16[] [0] ("values") _] -> w440
          frame "H" {
          }
          frame "L" {
          }
          frame "AUTO", Default {
          }
        }
        n205 = call "CODMnMB_api.vi"("STEP"=enum16{"open", "read", "write", "close"}."write", "values"=w440, "starting address"=u16 4276) -> ("error out"=w436:errorcluster)  [unwired: 6 in, 2 out]
      }
    }
  }
  n206 = Release Queue(queue=w4, error in (no error)=w3) -> ()  [unwired: 1 in, 3 out]
  n207 = Release Queue(queue=w9, error in (no error)=w8) -> ()  [unwired: 1 in, 3 out]
